vi "variantCtrlIoCalibPoints.vi"(4 "isRequired (T)":bool=TRUE, 6 "menu in (get)":enum16{"get", "set"}(ring), 8 "error in":errorcluster, 9 "calibration":T1[](array[typedef]) {"Y" format="%#.1f"}, 11 "variant in":variant) -> (0 "error out":errorcluster, 1 "UiCalibArray":T1[](array[typedef]) {"Y" format="%#.1f"}, 2 "found/replaced":bool, 3 "variant out":variant)   [LabVIEW 2024]
uses:
  controls/typeXyPoint.ctl
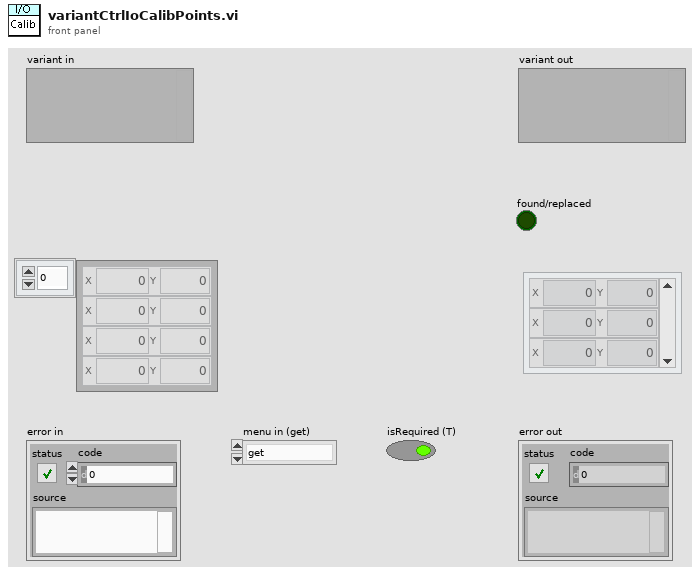
[diagram p1: front panel]
types:
  T1 = typedef "typeXyPoint.ctl" = cluster{"X":dbl, "Y":dbl}
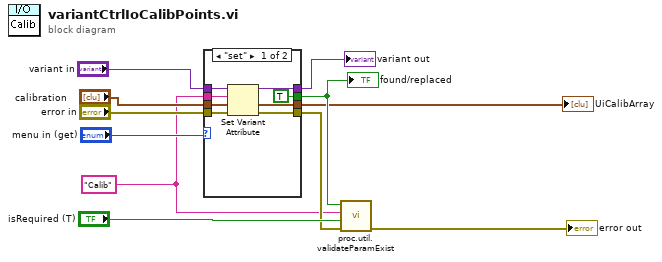
[diagram p0: block diagram]
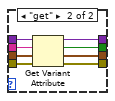
[diagram p2: hidden frame]
diagram:
  w1 = "Calib" ("String")
  n1 = case shown="\"set\"" "menu in (get)" {
    tunnel: "error in" -> [w18 w26]
    tunnel: "calibration" -> [w13 w25]
    tunnel: "variant in" -> [w17 w24]
    tunnel: [w16 w23] -> w5
    tunnel: [TRUE w22] -> w6
    tunnel: [w15 w21] -> w9
    tunnel: w1 -> [w14 w20]
    tunnel: [w13 w19] -> w2
    frame "set" {
      n2 = Set Variant Attribute(Variant=w17, name=w14, value=w13, error in=w18) -> (Variant out=w15:variant, error out=w16:errorcluster)  [unwired: 1 out]
    }
    frame "get" {
      n3 = Get Variant Attribute(Variant=w24, name=w20, default value (empty Variant)=w25, error in=w26) -> (duplicate Variant=w21:variant, found=w22:bool, value=w19:T1[], error out=w23:errorcluster)
    }
  }
  "found/replaced" <- w6
  "variant out" <- w9
  "UiCalibArray" <- w2
  n4 = call "proc.util.validateParamExist.vi"("error in"=w5, "isRequired"="isRequired (T)", "Param Label"=w1, "isFound"=w6) -> ("error out"=→"error out":errorcluster)  [unwired: 7 in]
